vi "Sub_Read_Variable_Header.vi"(8 "error in (no error)":errorcluster, 9 "QoS":T1(ring), 10 "Variable Header":u8[](array[numeric]) format="%x") -> (0 "error out":errorcluster, 1 "remaining bytes":u8[](array[numeric]) format="%x", 2 "Message ID":u16=1 format="%x", 3 "Topic Name":string="Topic")   [LabVIEW 2025, in "DAQIO MQTT.lvlib"]
uses:
  DAQIO MQTT.lvlib
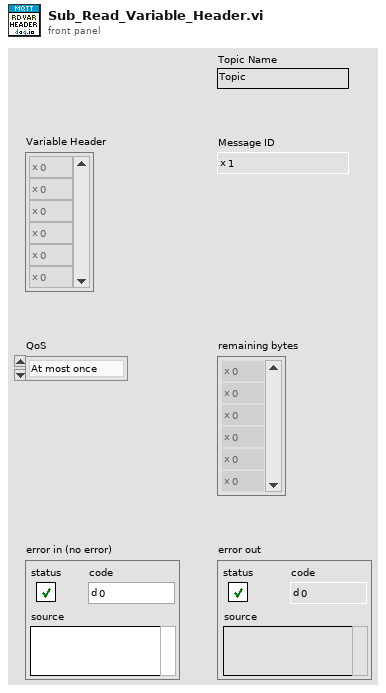
[diagram p1: front panel]
types:
  T1 = enum8{"At most once", "At least once", "Exactly once", "Reserved"}
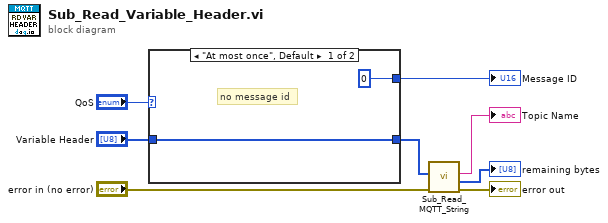
[diagram p0: block diagram]
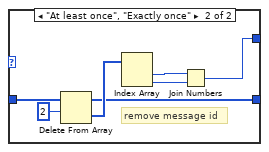
[diagram p2: hidden frame]
diagram:
  n1 = case shown="\"At most once\", Default" "QoS" {
    tunnel: "Variable Header" -> [w10 w17]
    tunnel: [w10 w12] -> w5
    tunnel: [u16 0 w11] -> w1
    frame "At most once", Default {
      # "no message id"
    }
    frame "At least once", "Exactly once" {
      # "remove message id"
      n2 = Delete From Array(array=w17, length=2) -> (deleted portion=w15:u8[], array with subset deleted=w12:u8[])  [unwired: 1 in]
      n3 = Index Array(array=w15) -> (element #1=w13:u8, element #2=w14:u8)  [unwired: 2 in]
      n4 = Join Numbers(hi=w13, lo=w14) -> ((hi.lo)=w11:u16)
    }
  }
  "Message ID" <- w1
  n5 = call "Sub_Read_MQTT_String.vi"("error in (no error)"="error in (no error)", "UTF8 Byte Array"=w5) -> ("error out"=→"error out":errorcluster, "remaining bytes"=→"remaining bytes":u8[], "String"=→"Topic Name":string)  [unwired: 7 in]
